vi "Stacking algorithm.vi"(0 "初始進入":bool[][](array[boolean]), 1 "Circles (Shape Detection 1) 2":T1(array[cluster]) {"Position"."Y" format="%.2f"; "Position"."X" format="%.2f"}, 5 "KNR in":T2, 11 "Error":errorcluster, 12 "ふ计":i32) -> (2 "底盤T數":i32, 3 "X":i32, 4 "最終堆疊版 2":bool[][](array[boolean]), 6 "KNR out":T2, 7 "Y軸補正":i32, 8 "旋轉數":i32, 10 "配對數":i32, 13 "層數":i32, 14 "Y":i32, 15 "error out":errorcluster)   [LabVIEW 2013]
uses:
  <userlib>/KNR OS 3.0 LabVIEW Toolkit/Type Definition/KNR3 Reference.ctl
  <userlib>/_FPGA Interface Advanced Tools/FPGA Interface Base/FPGA Interface Base.lvclass
  <userlib>/KNR OS 3.0 LabVIEW Toolkit/Type Definition/Resource.ctl
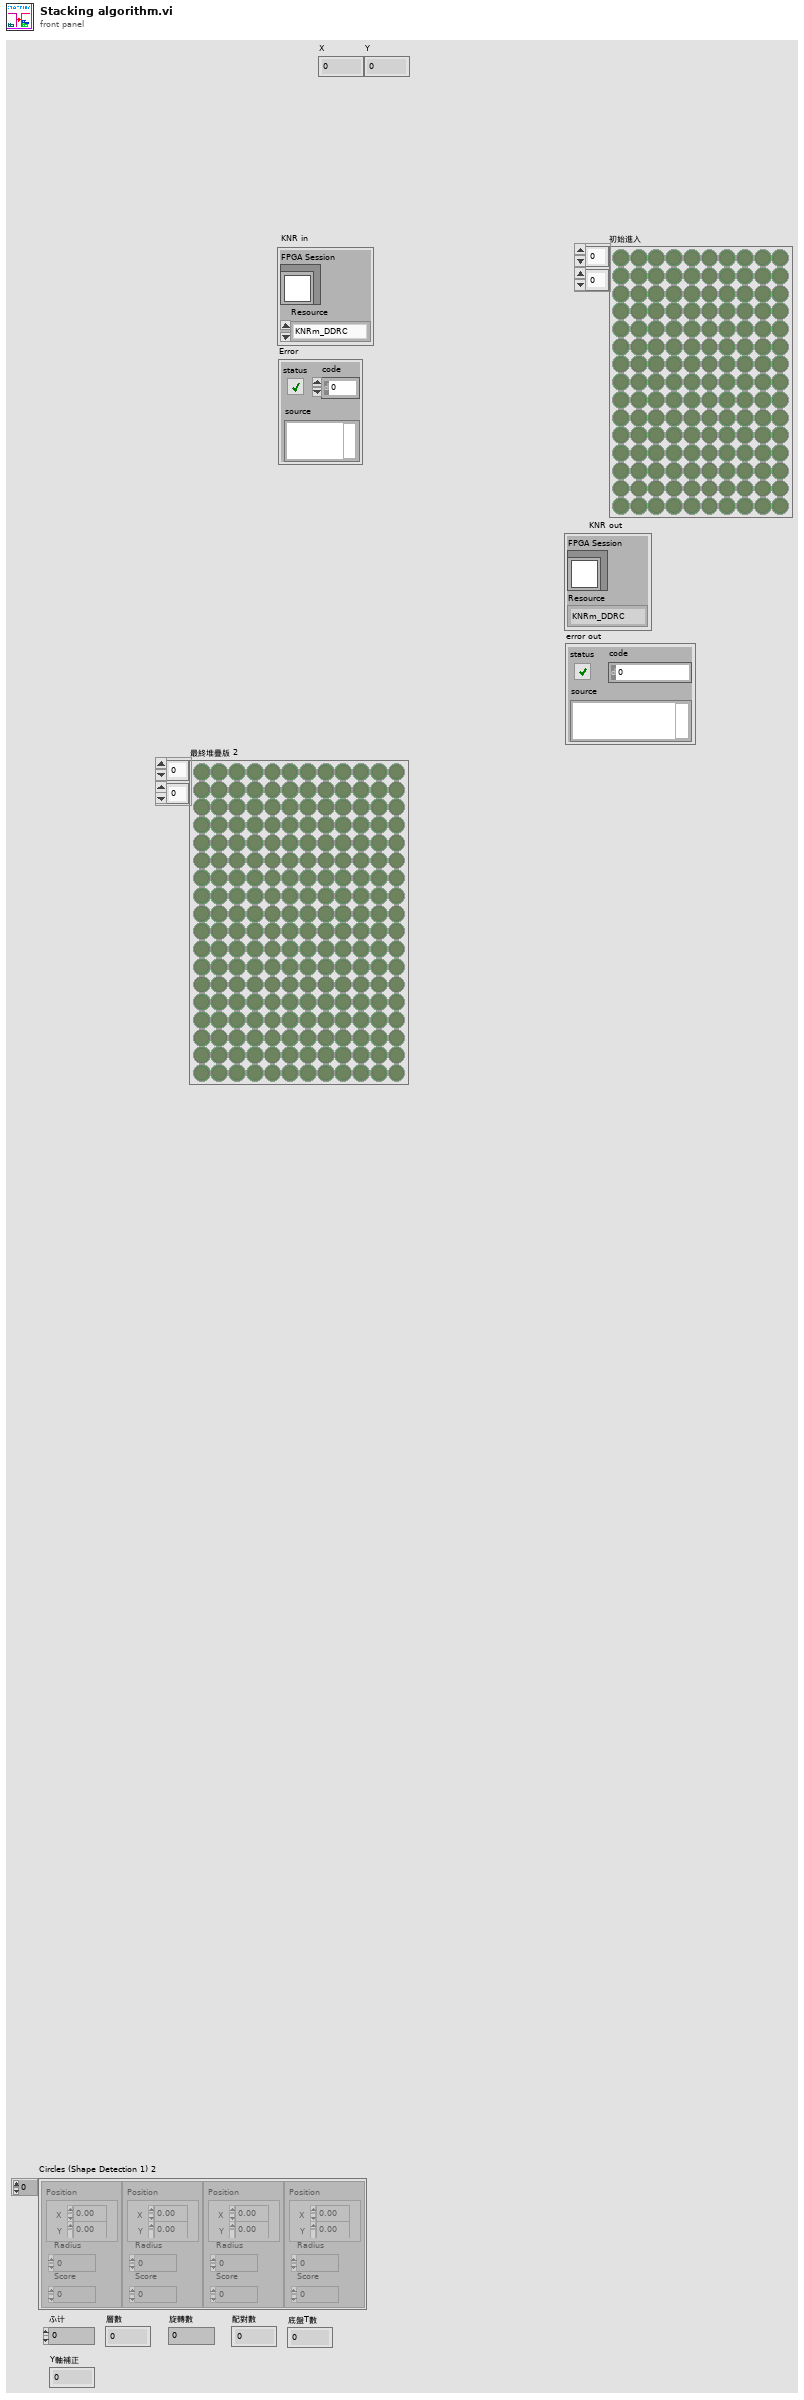
[diagram p1: front panel]
types:
  T1 = cluster{"Position":cluster{"X":sgl, "Y":sgl}, "Radius":dbl, "Score":dbl}[]
  T2 = typedef "KNR3 Reference.ctl" = cluster{"FPGA Session":refnum<class "FPGA Interface Base.lvclass">, "Resource":T3}
  T3 = typedef "Resource.ctl" = enum16{"KNRm_DDRC", "KNRm_DDDD", "KNRm_DDDR", "KNRm_DDDC", "KNR"}
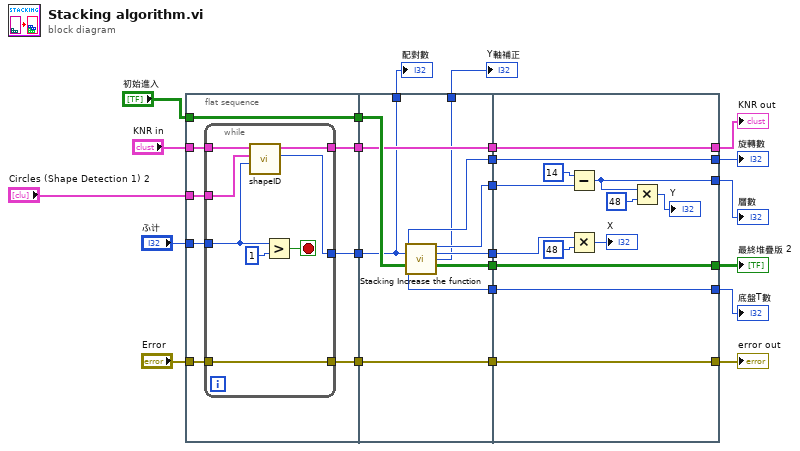
[diagram p0: block diagram]
diagram:
  n1 = flat-sequence {
    tunnel: [w32] -> w24
    tunnel: "初始進入" -> [w31]
    tunnel: [w31] -> w21
    tunnel: "KNR in" -> [w30]
    tunnel: "Error" -> [w29]
    tunnel: [w28] -> w18
    tunnel: "Circles (Shape Detection 1) 2" -> [w27]
    tunnel: "ふ计" -> [w26]
    tunnel: [w25] -> w7
    tunnel: w24 -> [w45]
    tunnel: w21 -> [w50]
    tunnel: w18 -> [w46]
    tunnel: [w49] -> w17
    tunnel: [w48] -> w16
    tunnel: [w47] -> w15
    tunnel: [w46] -> w11
    tunnel: [w45] -> w9
    tunnel: w7 -> [w44]
    tunnel: [w44] -> w6
    tunnel: [w43] -> w4
    tunnel: [w42] -> w2
    tunnel: [w41] -> w1
    tunnel: [w63] -> w23
    tunnel: w17 -> [w63]
    tunnel: w16 -> [w62]
    tunnel: w15 -> [w58]
    tunnel: [w55] -> w12
    tunnel: w11 -> [w55]
    tunnel: [w52] -> w10
    tunnel: [w54] -> w8
    tunnel: w6 -> [w54]
    tunnel: [w53] -> w5
    tunnel: w4 -> [w53]
    tunnel: [w51] -> w3
    tunnel: w2 -> [w51]
    frame #0 {
      n2 = while {
        tunnel: [w36] -> w32
        tunnel: w30 -> [w38]
        tunnel: w29 -> [w33]
        tunnel: [w37] -> w28
        tunnel: w27 -> [w35]
        tunnel: w26 -> [w34]
        tunnel: [w33] -> w25
        stop <- w40 stop-if-true
        n3 = call "shapeID.vi"("Nb Circles (Circle Detection 1)"=w34, "Circles (Shape Detection 1)"=w35, "KNR in"=w38) -> ("配對數"=w36:i32, "KNR out"=w37:T2)  [unwired: 5 in, 2 out]
        n4 = Greater?(x=w34, y=1) -> (0:w40:bool)
      }
    }
    frame #1 {
      n5 = call "Stacking Increase the function.vi"("積木種類"=w45, "初始進入"=w50) -> ("旋轉數"=w43:i32, "end"=w47:i32, "移動位置"=w48:i32, "Y軸補正"=w41:i32, "最終堆疊版"=w49:bool[][], "底盤T數"=w42:i32)  [unwired: 5 in, 3 out]
    }
    frame #2 {
      n6 = Subtract(x=14, y=w58) -> (x-y=w52:i32)
      n7 = Multiply(x=w62, y=48) -> (x*y=→"X":i32)
      n8 = Multiply(x=w52, y=48) -> (x*y=→"Y":i32)
    }
  }
  "最終堆疊版 2" <- w23
  "KNR out" <- w12
  "error out" <- w8
  "層數" <- w10
  "配對數" <- w9
  "旋轉數" <- w5
  "底盤T數" <- w3
  "Y軸補正" <- w1
